vi "FFT Power Spectrum.vi"   [LabVIEW 2016, in "xy_utilities.lvlib"]
doc: "Computes a Power Spectrum.\n\nWire data to the data input to determine the polymorphic instance to use or manually select the instance."
uses:
  xy_utilities.lvlib
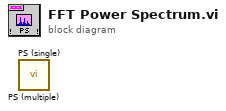
[diagram p0: block diagram]
diagram:
  n1 = call "PS (multiple).vi"() -> ()  [unwired: 9 in, 3 out]
  n2 = call "PS (single).vi"() -> ()  [unwired: 9 in, 3 out]
